vi "Example - Alignment (Grid).vi"() -> ()   [LabVIEW 2012]
doc: "This example shows how to use the UI Tools Alignment primitives to snap GObjects relative to some other GObject."
panel:
  in  "Offset":i16=10 min=-10 max=50 step=1
  in  "Border":i16 min=0 max=50 step=1
  in  "Width":i16=48 min=1 max=500 step=1
  in  "Cluster":cluster{"Move":bool}
  # "Set BUTTON \"AAA\" to TRUE to have the button follow the mouse cursor and snap on cluster grid.\nSet BUTTON \"AAA\" to FALSE to have the \"Object\" stay in that position."
  # "Adjust the parameters to create the grid as shown on the right.\n\n*You can use any GObject as the container or terminal to move."
  # "Rectangle"
  # "Offset"
  # "border"
  # "border"
  # "Offset"
  # "Width"
  # "Width"
  # "border"
  # "border"
  # "Width"
  # "Width"
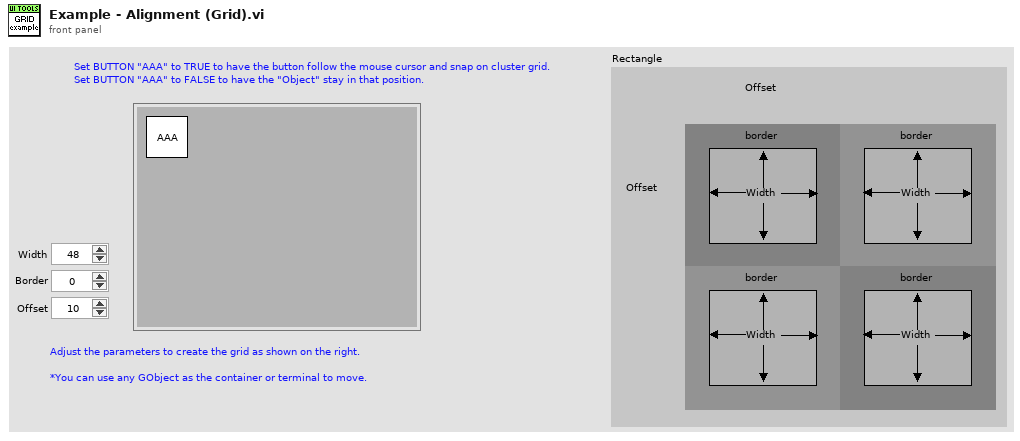
[diagram p1: front panel]
types:
  T1 = enum32{"invalid app kind", "Development System", "Run Time System", "Student Edition", "Embedded LabVIEW", "Evaluation", "Custom"}
  T2 = typedef "LVPoint32TypeDef.ctl" = cluster{"Horizontal":i32, "Vertical":i32}
  T3 = cluster{"left":i16, "top":i16, "right":i16, "bottom":i16}
  T4 = cluster{"left":i16, "top":i16, "right":i16, "bottom":i16}[][]
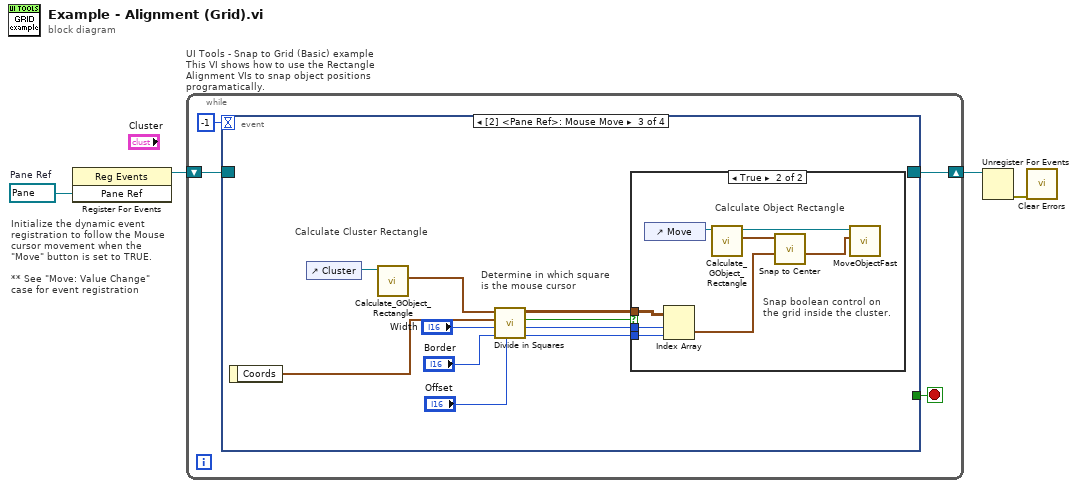
[diagram p0: block diagram]
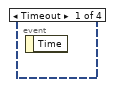
[diagram p2: hidden frame]
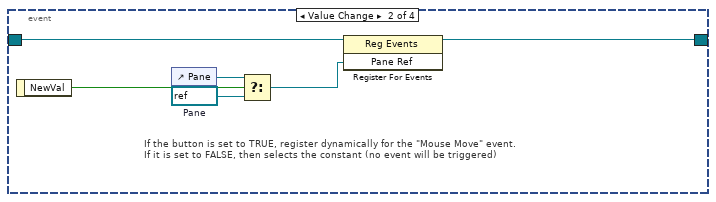
[diagram p3: hidden frame]
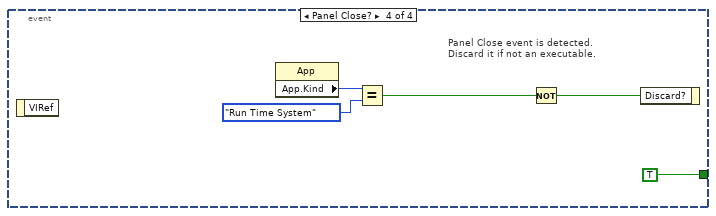
[diagram p5: hidden frame]
diagram:
  w3 = refnum<vi> refnum  # Pane Ref
  # "Initialize the dynamic event\nregistration to follow the Mouse\ncursor movement when the\n\"Move\" button is set to TRUE.\n\n** See \"Move: Value Change\"\ncase for event registration"
  n1 = register-events(w3) -> (reference out=w4:refnum<event-registration>)  [unwired: 2 in, 1 out]
  n2 = while "UI Tools - Snap to Grid (Basic) example\nThis VI shows how to use the Rectangle Alignment VIs to snap object positions programatically." {
    shift-right: [w5] -> w2
    shift-left: w4 -> [w6]
    stop <- w7 stop-if-true
    n3 = event shown="[2] <Pane Ref>: Mouse Move" {
      selector: w6 -> [_ w12 _ _]
      dyn-events: [_ w10 _ _] -> w5
      timeout: -1 -> [_ _ _ _]
      tunnel: [_ _ _ TRUE ("Discard?")] -> w7
      event Timeout {
        n4 = event-data() -> ()  [unwired: 2 out]
      }
      event "Cluster.Move": Value Change {
        w13 = refnum<vi> refnum  # Pane
        # "If the button is set to TRUE, register dynamically for the \"Mouse Move\" event.\nIf it is set to FALSE, then selects the constant (no event will be triggered)"
        n5 = event-data() -> ("NewVal"=w9:bool)  [unwired: 1 out]
        n6 = control-ref of="Pane"() -> (w14:refnum<vi>)
        n7 = Select(t=w14, s=w9, f=w13) -> (s? t:f=w11:refnum<vi>)
        n8 = register-events(reference=w12, w11) -> (reference out=w10:refnum<event-registration>)  [unwired: 1 in, 1 out]
      }
      event Mouse Move {
        # "Determine in which square\nis the mouse cursor"
        # "Calculate Cluster Rectangle"
        n9 = event-data() -> ("Coords"=w24:T2)  [unwired: 1 out]
        n10 = control-ref of="Cluster"() -> (w20:refnum<vi>)
        n11 = call "Calculate_GObject_Rectangle.vi"("GObject ref"=w20) -> ("Rectangle"=w19:T3)  [unwired: 2 in, 8 out]
        n12 = call "Divide in Squares.vi"("Offset (0)"="Offset", "Border (2)"="Border", "Width (48)"="Width", "Coords"=w24, "Rectangle"=w19) -> ("Column"=w22:i32, "Row"=w21:i32, "in squares?"=w18:bool, "Zones Rectangles"=w23:T4)  [unwired: 3 out]
        n13 = case shown="True" w18 {
          tunnel: w23 -> [_ w30]
          tunnel: w22 -> [_ w29]
          tunnel: w21 -> [_ w28]
          frame False {
          }
          frame True {
            # "Calculate Object Rectangle"
            # "Snap boolean control on\nthe grid inside the cluster."
            n14 = control-ref of="Move"() -> (w32:refnum<vi>)
            n15 = Index Array(array=w30, index (row)=w28, index (col)=w29) -> (element=w26:T3)
            n16 = call "Calculate_GObject_Rectangle.vi"("GObject ref"=w32) -> ("Rectangle"=w27:T3, "GObject ref dup"=w31:refnum<vi>)  [unwired: 2 in, 7 out]
            n17 = call "Snap to Center.vi"("Fixed Rect"=w26, "Rect"=w27) -> ("TopLeft point"=w25:cluster{"x":i32, "y":i32})  [unwired: 9 out]
            n18 = call "MoveObjectFast.vi"("Position"=w25, "GObj Refnum"=w31) -> ()  [unwired: 1 in, 9 out]
          }
        }
      }
      event Panel Close? {
        # "Panel Close event is detected.\nDiscard it if not an executable."
        n19 = event-data() -> ()  [unwired: 2 out]
        n20 = property class="App"() -> ("App.Kind"=w36:T1)  [unwired: 2 in, 2 out]
        n21 = Equal?(x=w36, y=T1."Run Time System" ("Application:Kind")) -> (x = y?=w35:bool)
        n22 = Not(x=w35) -> (.not. x?=w33:bool)
        n23 = event-data("Discard?"=w33) -> ()  [unwired: 1 in, 1 out]
      }
    }
  }
  n24 = Unregister For Events(event registration refnum=w2) -> (error out=w1:errorcluster)  [unwired: 1 in]
  n25 = call <vilib>:"Clear Errors.vi"("error in (no error)"=w1) -> ()  [unwired: 7 out]
